vi "NET-RX UDP Service.vi"(7 "Max Rx Byte Size":i32=10000, 8 "Module ID":i32=-1, 9 "Caller MsgQ":refnum<class "DQMH-GenNet Message Queue.lvclass">, 10 "Stop Module":refnum<user-event>, 11 "UDP Connection ID":refnum<k16>) -> ()   [LabVIEW 2020, in "GenNet-Client.lvlib"]
doc: "____\nHAMPEL SOFTWARE ENGINEERING v3.8.0 (2023-12-18 14:41)"
uses:
  GenNet-Client.lvlib
  DQMH-GenNet Message Queue.lvclass
  C:/Program Files (x86)/National Instruments/LabVIEW 2020/vi.lib/Delacor/Delacor QMH/Libraries/Message Queue_class/Delacor_lib_QMH_Message Queue.lvclass
  GenNet-Server/Stop Argument--cluster.ctl
  <vilib>/Delacor/Delacor QMH/Libraries/Message Queue_class/Delacor_lib_QMH_Message Queue.lvclass/Delacor_lib_QMH_Message Queue.ctl
  <vilib>/Delacor/Delacor QMH/Libraries/Message Queue_class/Delacor_lib_QMH_Enqueue Message (Single).vi
  GenNet Version-Safe Unflatten Variant.vi
  <vilib>/Delacor/Delacor QMH/Libraries/Message Queue_class/Delacor_lib_QMH_Message Queue.lvclass
  hse-gennet.lvlib
  C:/GitLab-Runner/builds/7NHnU7RQc/0/open-source/hse-libraries/Source/hse-gennet/DQMH-GenNet Message Queue.lvclass
  GenNet-Server/GenNet-Server.lvlib
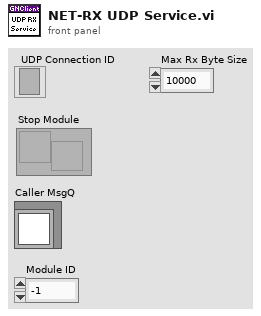
[diagram p1: front panel]
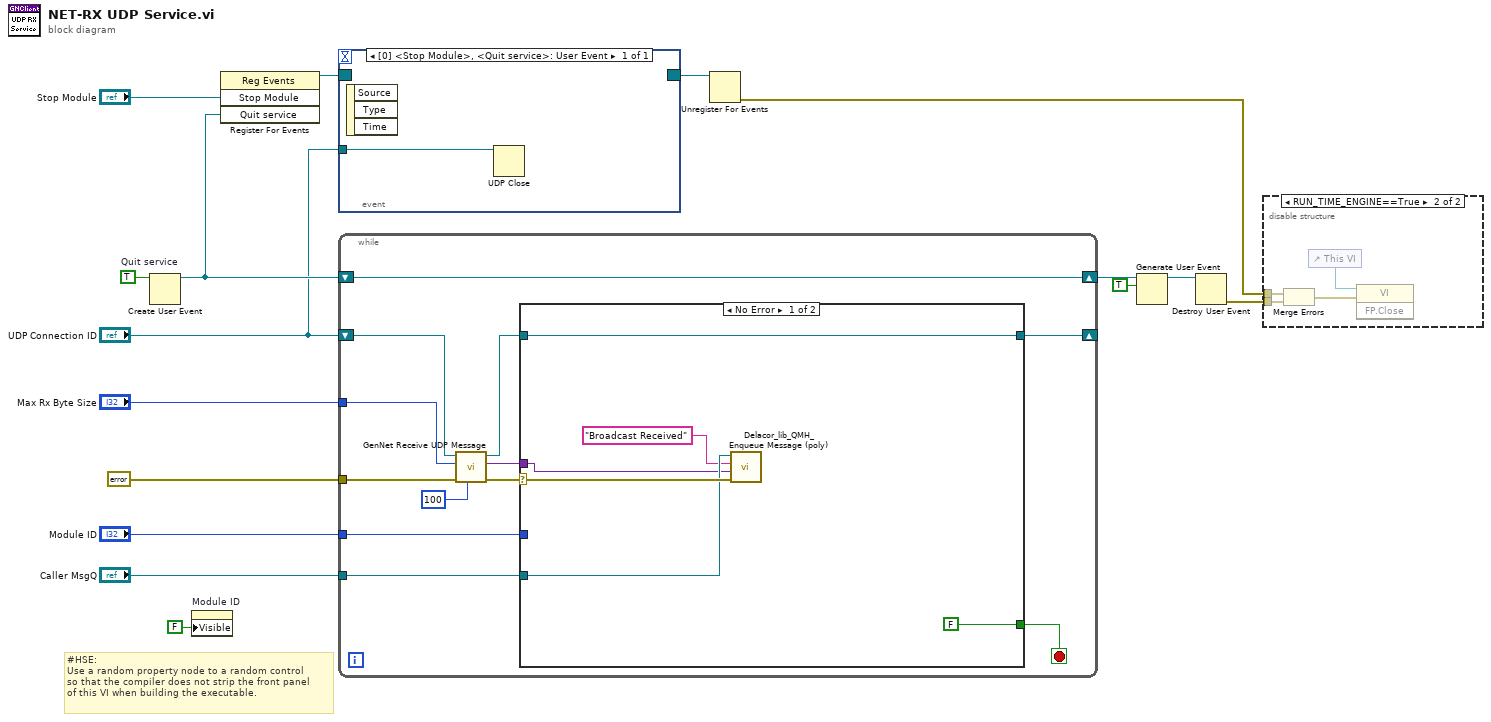
[diagram p0: block diagram]
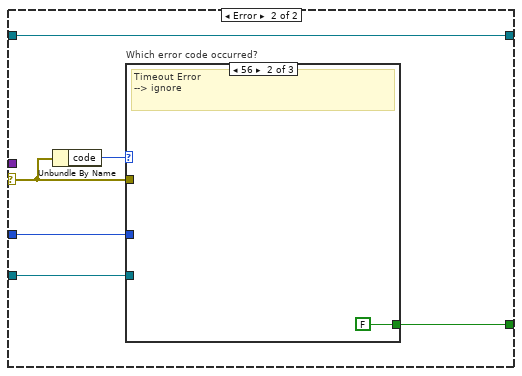
[diagram p3: hidden frame]
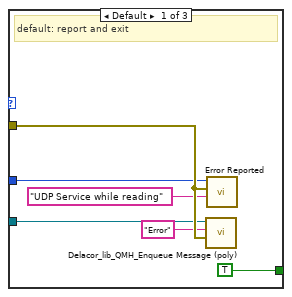
[diagram p4: hidden frame]
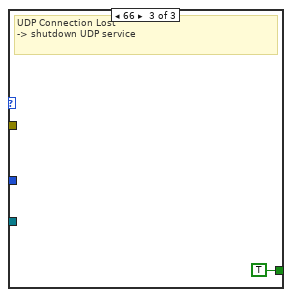
[diagram p5: hidden frame]
diagram:
  w11 = TRUE  # Quit service
  # "#HSE: \nUse a random property node to a random control \nso that the compiler does not strip the front panel \nof this VI when building the executable."
  n1 = Create User Event(user event datatype=w11) -> (user event=w12:refnum<user-event>)  [unwired: 1 in, 1 out]
  n2 = property on="Module ID" class="DigNum (strict)"("Visible"=FALSE) -> ()  [unwired: 2 in, 2 out]
  n3 = register-events("Stop Module", w12) -> (reference out=w10:refnum<event-registration>)  [unwired: 2 in, 1 out]
  n4 = event shown="[0] <Stop Module>, <Quit service>: User Event" {
    selector: w10 -> [_]
    dyn-events: [_] -> w16
    timeout: _ -> [_]
    tunnel: "UDP Connection ID" -> [w17]
    event User Event {
      n5 = event-data() -> ()  [unwired: 1 in, 3 out]
      n6 = UDP Close(connection ID=w17) -> ()  [unwired: 1 in, 2 out]
    }
  }
  n7 = while {
    shift-right: [w29] -> _
    shift-left: "UDP Connection ID" -> [w20]
    tunnel: errorcluster {"status"=FALSE, "code"=0, "source"=""} ("error out") -> [w24]
    shift-right: [w28] -> w13
    shift-left: w12 -> [w28]
    tunnel: "Module ID" -> [w26]
    tunnel: "Caller MsgQ" -> [w25]
    tunnel: "Max Rx Byte Size" -> [w18]
    stop <- w27 stop-if-true
    n8 = call "GenNet Receive UDP Message.vi"("timeout [ms]"=100, "error in (no error)"=w24, "Max Byte Size"=w18, "UDP Network Connection in"=w20) -> ("error out"=w23:errorcluster, "Message Data"=w22:variant, "UDP Network Connection out"=w21:refnum<k16>)  [unwired: 5 in]
    n9 = case shown="No Error" w23 {
      selector: w23 -> [w34 w39]
      tunnel: w21 -> [w32 w37]
      tunnel: [w32 w37] -> w29
      tunnel: [FALSE w36] -> w27
      tunnel: w26 -> [_ w38]
      tunnel: w25 -> [w33 w40]
      tunnel: w22 -> [w31 _]
      frame No Error {
        n10 = call-poly <vilib>:"Delacor_lib_QMH_Enqueue Message (poly).vi"("error in"=w34, "Message Data"=w31, "Message"="Broadcast Received", "Message Queue in"=w33) -> ()  [unwired: 6 in, 2 out]
      }
      frame Error {
        n11 = Unbundle By Name(w39) -> ("code"=w41:i32)
        n12 = case "Which error code occurred?" shown="56" w41 {
          tunnel: w40 -> [w45 _ _]
          tunnel: w39 -> [w47 _ _]
          tunnel: w38 -> [w44 _ _]
          tunnel: [TRUE FALSE TRUE] -> w36
          frame Default {
            # "default: report and exit"
            n13 = call-poly <vilib>:"Delacor_lib_QMH_Enqueue Message (poly).vi"("Message Data"=w47, "Message"="Error", "Message Queue in"=w45) -> ()  [unwired: 7 in, 2 out]
            n14 = call "Error Reported.vi"("Additional Information"="UDP Service while reading", "Error"=w47, "Module ID"=w44) -> ()  [unwired: 8 in, 1 out]
          }
          frame 56 {
            # "Timeout Error\n--> ignore"
          }
          frame 66 {
            # "UDP Connection Lost\n-> shutdown UDP service"
          }
        }
      }
    }
  }
  n15 = Unregister For Events(event registration refnum=w16) -> (error out=w4:errorcluster)  [unwired: 1 in]
  n16 = Generate User Event(user event=w13, event data cluster=TRUE ("event data")) -> (user event out=w15:refnum<user-event>)  [unwired: 2 in, 1 out]
  n17 = Destroy User Event(user event=w15) -> (error out=w5:errorcluster)  [unwired: 1 in]
  n18 = disable-structure shown="RUN_TIME_ENGINE==True" {
    disable-tunnel: w5 -> [_ w51]
    disable-tunnel: w4 -> [_ w50]
    frame condition #0 (active) {
    }
    frame condition #1 {
      n19 = Merge Errors(w50, w51) -> (w52:errorcluster)
      n20 = control-ref of="This VI"() -> (w53:refnum<vi>)
      n21 = invoke class="VI" method="FP.Close"(reference=w53, error in=w52) -> ()  [unwired: 1 in, 3 out]
    }
  }
